vi "Child Text.vi"(8 "Error In":errorcluster, 11 "Bookmark":T1) -> (0 "Error Out":errorcluster, 3 "Child Text":string[](array[string]))   [LabVIEW 2018, in "Bookmark Manager.lvlib"]
uses:
  Bookmark Manager.lvlib
  Controls/BMark_Bookmark Data.ctl
  Controls/BMark_VI_Identifier.ctl
  <vilib>/addons/analyzer/_analyzerctrls.llb/VIAnCtl Analysis App Info.ctl
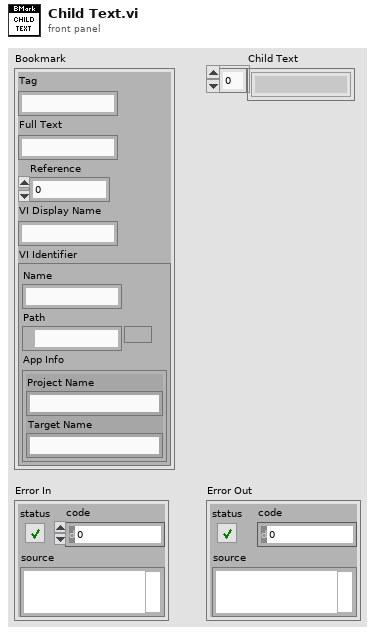
[diagram p1: front panel]
types:
  T1 = typedef "Bookmark Manager.lvlib/BMark_Bookmark Data.ctl" = cluster{"Tag":string, "Full Text":string, "Reference":i32, "VI Display Name":string, "VI Identifier":T2}
  T2 = typedef "Bookmark Manager.lvlib/BMark_VI_Identifier.ctl" = cluster{"Name":string, "Path":path, "App Info":T3}
  T3 = typedef "VIAnCtl Analysis App Info.ctl" = cluster{"Project Name":string, "Target Name":string}
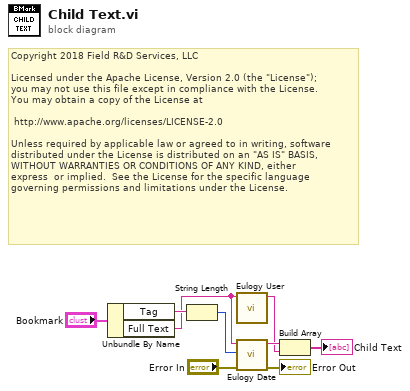
[diagram p0: block diagram]
diagram:
  # "Copyright 2018 Field R&D Services, LLC\n\nLicensed under the Apache License, Version 2.0 (the \"License\");\nyou may not use this file except in compliance with the License.\nYou may obtain a copy of the License at\n\n\thttp://www.apache.org/licenses/LICENSE-2.0\n\nUnless required by applicable law or agreed to in writing, software\ndistributed under the License is distributed on an \"AS IS\" BASIS,\nWITHOUT WARRANTIES OR CONDITIONS OF ANY KIND, either \nexpress  or implied.  See the License for the specific language \ngoverning permissions and limitations under the License."
  n1 = Unbundle By Name("Bookmark") -> ("Tag"=w2:string, "Full Text"=w1:string)
  n2 = String Length(string=w2) -> (length=w9:i32)
  n3 = call "Eulogy User.vi"("Label Text"=w1) -> ("User"=w5:string)  [unwired: 10 in]
  n4 = call "Eulogy Date.vi"("Error In"="Error In", "Tag Length"=w9, "Label Text"=w1) -> ("Error Out"=→"Error Out":errorcluster, "Date"=w8:string)  [unwired: 7 in]
  n5 = Build Array(w8, w5) -> (→"Child Text":string[])
